vi "Git Version Info.vi"(8 "error in":errorcluster, 11 "Config Manager in":refnum<class "Config Manager Class.lvclass">) -> (0 "error out":errorcluster, 2 "Git Data":string, 3 "Config Manager out":refnum<class "Config Manager Class.lvclass">)   [LabVIEW 2017, in "Config Manager Class.lvclass"]
uses:
  Config Manager Class.lvclass
  Config Manager Class.lvclass/Config Manager Class.ctl
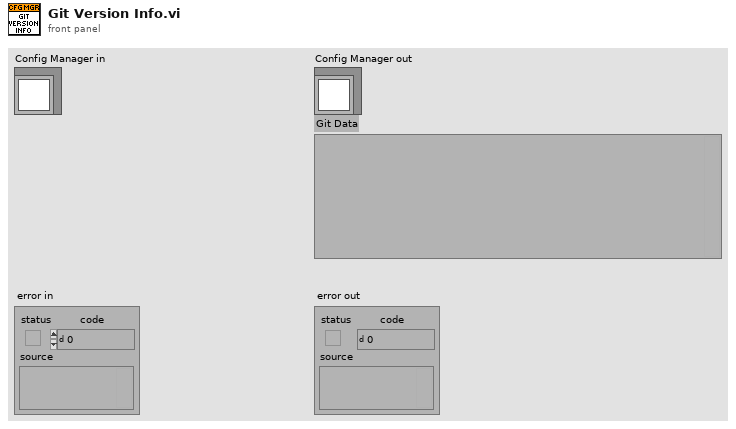
[diagram p1: front panel]
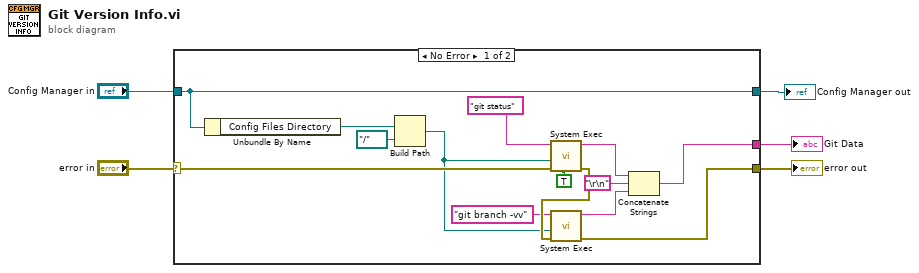
[diagram p0: block diagram]
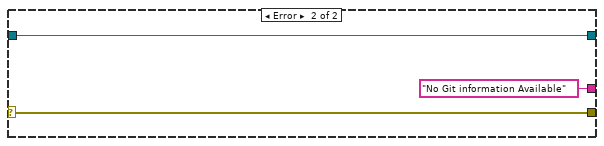
[diagram p2: hidden frame]
diagram:
  n1 = case shown="No Error" "error in" {
    selector: "error in" -> [w17 w21]
    tunnel: [w10 "No Git information Available" ("standard output")] -> w5
    tunnel: [w11 w21] -> w4
    tunnel: "Config Manager in" -> [w7 w20]
    tunnel: [w7 w20] -> w1
    frame No Error {
      n2 = Unbundle By Name(w7) -> ("Config Files Directory"=w6:path)
      n3 = Build Path(base path=w6, name or relative path=path "../..") -> (appended path=w9:path)
      n4 = call <vilib>:"System Exec.vi"("run minimized? (F)"=TRUE, "error in (no error)"=w17, "working directory"=w9, "command line"="git status") -> ("error out"=w16:errorcluster, "standard output"=w13:string)  [unwired: 4 in, 2 out]
      n5 = call <vilib>:"System Exec.vi"("error in (no error)"=w16, "working directory"=w9, "command line"="git branch -vv") -> ("error out"=w11:errorcluster, "standard output"=w12:string)  [unwired: 5 in, 2 out]
      n6 = Concatenate Strings(w13, "\r\n", w12) -> (w10:string)
    }
    frame Error {
    }
  }
  "Git Data" <- w5
  "error out" <- w4
  "Config Manager out" <- w1
